vi "LabVIEW IV 2주차.vi"() -> ()   [LabVIEW 2015]
uses:
  <vilib>/Analysis/1siggen.llb/Ramp Pattern by Samples.vi
  <vilib>/Analysis/NI_AALBase.lvlib
panel:
  in  "Start":bool
  in  "Both forward & backward sweep":bool=TRUE
  in  "VISA resource name":refnum<visa-resource-name>="GPIB0::15::INSTR"
  in  "stop":bool
  in  "samples":i32=128
  in  "Voltage End":dbl=1.0
  in  "Voltage start":dbl
  out "XY Graph":cluster{"Y":dbl[], "Y":dbl[]}[](graph)
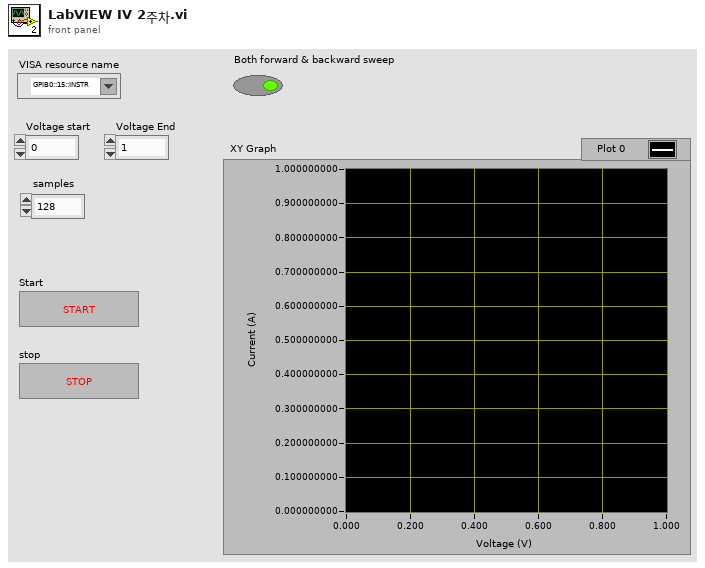
[diagram p1: front panel]
types:
  T1 = enum16{"open", "replace", "create", "open or create", "replace or create", "replace or create with confirmation"}
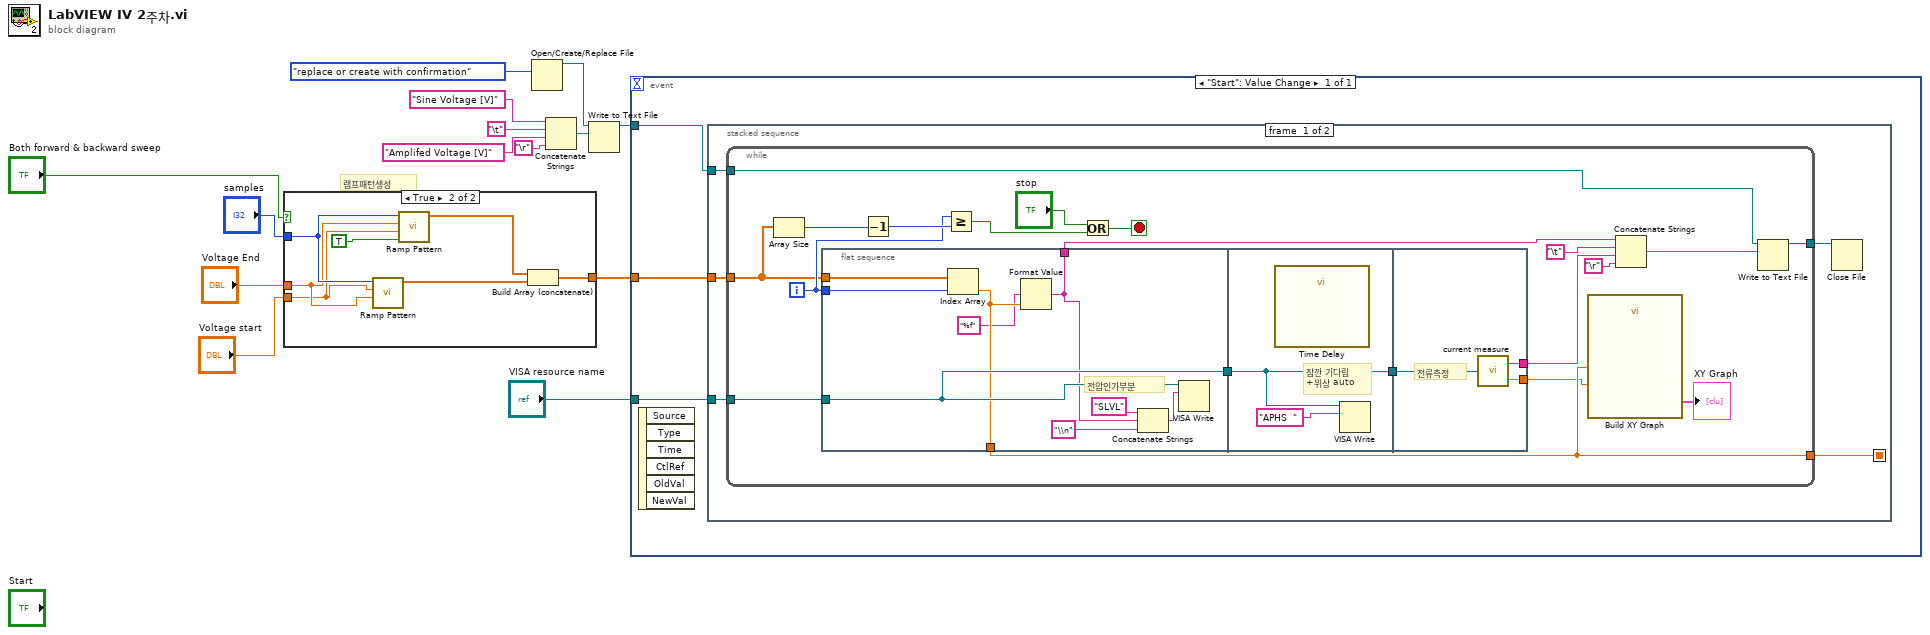
[diagram p0: block diagram]
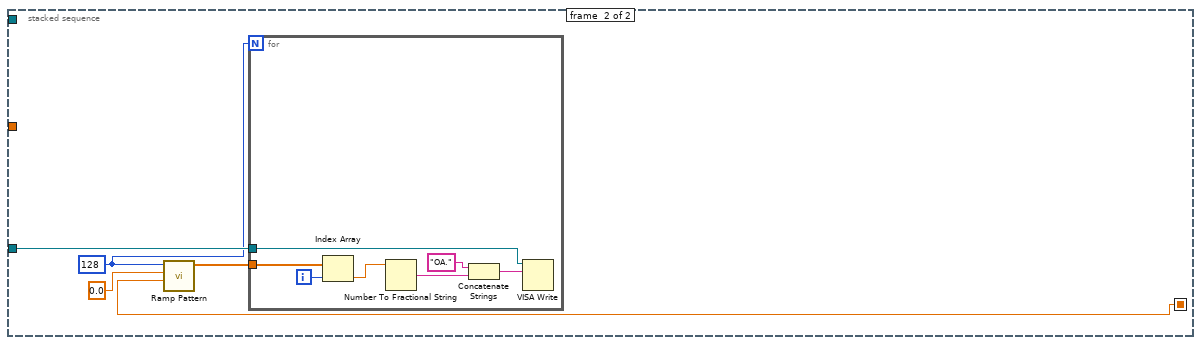
[diagram p2: hidden frame]
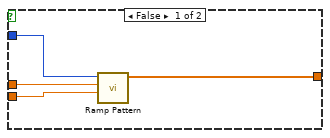
[diagram p3: hidden frame]
diagram:
  # "램프패턴생성"
  n1 = case shown="True" "Both forward & backward sweep" {
    tunnel: "Voltage start" -> [w18 w19]
    tunnel: "Voltage End" -> [w17 w20]
    tunnel: [w16 w21] -> w12
    tunnel: "samples" -> [w15 w25]
    frame False {
      n2 = call-poly <vilib>:"Ramp Pattern.vi"("start"=w18, "end"=w17, "samples"=w15) -> ("Ramp Pattern"=w16:dbl[])  [unwired: 7 in, 1 out]
    }
    frame True {
      n3 = call-poly <vilib>:"Ramp Pattern.vi"("start"=w20, "end"=w19, "samples"=w25) -> ("Ramp Pattern"=w22:dbl[])  [unwired: 7 in, 1 out]
      n4 = call-poly <vilib>:"Ramp Pattern.vi"("exclude end?"=TRUE, "start"=w19, "end"=w20, "samples"=w25) -> ("Ramp Pattern"=w23:dbl[])  [unwired: 6 in, 1 out]
      n5 = Build Array (concatenate)(w23, w22) -> (w21:dbl[])
    }
  }
  n6 = Open/Create/Replace File(operation (0:open)=T1."replace or create with confirmation") -> (refnum out=w9:refnum<file>)  [unwired: 5 in, 2 out]
  n7 = Concatenate Strings("Sine Voltage [V]" ("string"), "\t", "Amplifed Voltage [V]" ("string"), "\r") -> (w6:string)
  n8 = Write to Text File(file (use dialog)=w9, text=w6) -> (refnum out=w3:refnum<file>)  [unwired: 2 in, 2 out]
  n9 = event shown="[0] \"Start\": Value Change" {
    selector: _ -> [_]
    dyn-events: _ -> [_]
    timeout: _ -> [_]
    tunnel: w12 -> [w28]
    tunnel: w3 -> [w27]
    tunnel: "VISA resource name" -> [w26]
    event "Start": Value Change {
      n10 = event-data() -> ()  [unwired: 1 in, 6 out]
      n11 = stacked-sequence {
        seq-local: [w29 _] -> [_ w71]
        tunnel: w28 -> [w33 _]
        tunnel: w27 -> [w31 _]
        tunnel: w26 -> [w30 w69]
        frame #0 {
          n12 = while {
            tunnel: w33 -> [w38]
            tunnel: w31 -> [w48]
            tunnel: [w47] -> w32
            tunnel: w30 -> [w41]
            tunnel: [w35] -> w29
            i -> [w49]
            stop <- w36 stop-if-true
            n13 = Array Size(array=w38) -> (size(s)=w37:i32)
            n14 = flat-sequence {
              tunnel: w38 -> [w62]
              tunnel: w49 -> [w61]
              tunnel: [w57] -> w35
              tunnel: [w56] -> w46
              tunnel: w41 -> [w58]
              tunnel: [w58] -> w39
              tunnel: [w64] -> w40
              tunnel: w39 -> [w64]
              tunnel: [w66] -> w45
              tunnel: w40 -> [w67]
              tunnel: [w65] -> w34
              frame #0 {
                # "전압인가부분"
                n15 = Index Array(array=w62, index=w61) -> (element=w57:dbl)
                n16 = Format Value(format string="%f" ("write buffer"), value (0)=w57) -> (output string=w56:string)  [unwired: 1 in]
                n17 = Concatenate Strings("SLVL" ("write buffer"), w56, "\\n" ("write buffer")) -> (w60:string)
                n18 = VISA Write(VISA resource name=w58, write buffer=w60) -> ()  [unwired: 1 in, 3 out]
              }
              frame #1 {
                # "잠깐 기다림\n+위상 auto"
                n19 = call "Time Delay"() -> ()  [unwired: 11 in, 1 out]
                n20 = VISA Write(VISA resource name=w64, write buffer="APHS  ") -> ()  [unwired: 1 in, 3 out]
              }
              frame #2 {
                # "전류측정"
                n21 = call "current measure.vi"("VISA Refnum in"=w67) -> ("read buffer"=w66:string, "Numeric"=w65:dbl)
              }
            }
            n22 = Decrement(x=w37) -> (x-1=w52:i32)
            n23 = Greater Or Equal?(x=w49, y=w52) -> (x >= y?=w50:bool)
            n24 = Or(x="stop", y=w50) -> (x .or. y?=w36:bool)
            n25 = call "Build XY Graph"("Y Input"=w34, "X Input"=w35) -> ("XY Graph"=→"XY Graph":cluster{"X":dbl[], "Y":dbl[]}[])  [unwired: 8 in, 1 out]
            n26 = Concatenate Strings(w46, "\t", w45, "\r") -> (w42:string)
            n27 = Write to Text File(file (use dialog)=w48, text=w42) -> (refnum out=w47:refnum<file>)  [unwired: 2 in, 2 out]
          }
          n28 = Close File(refnum=w32) -> ()  [unwired: 1 in, 2 out]
        }
        frame #1 {
          w68 = 128 ("samples")
          n29 = call-poly <vilib>:"Ramp Pattern.vi"("start"=w71, "end"=0.0, "samples"=w68) -> ("Ramp Pattern"=w70:dbl[])  [unwired: 7 in, 1 out]
          n30 = for {
            N: w68 -> [_]
            tunnel: w70 -> [w76]
            tunnel: w69 -> [w77]
            i -> [w75]
            n31 = Index Array(array=w76, index=w75) -> (element=w74:dbl)
            n32 = Number To Fractional String(number=w74) -> (F-format string=w73:string)  [unwired: 3 in]
            n33 = Concatenate Strings("OA." ("write buffer"), w73) -> (w78:string)
            n34 = VISA Write(VISA resource name=w77, write buffer=w78) -> ()  [unwired: 1 in, 3 out]
          }
        }
      }
    }
  }
